vi "Create Resources.vi"(0 "reference fpga in":refnum<class "niUSRP Reference FPGA v1.lvclass">) -> (4 "reference fpga out":refnum<class "niUSRP Reference FPGA v1.lvclass">)   [LabVIEW 2025, in "niUSRP Reference FPGA v1.lvclass"]
uses:
  niUSRP Reference FPGA v1.lvclass
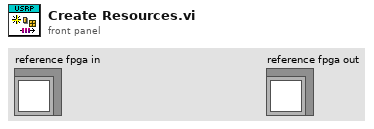
[diagram p1: front panel]
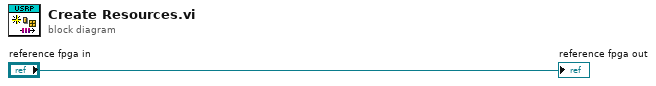
[diagram p0: block diagram]
diagram:
  "reference fpga out" <- "reference fpga in"
